vi "Set Controls.vi"(8 "error in (no error)":errorcluster, 9 "data values":variant[](array[variant]), 10 "control indexes":i32[](array[numeric]), 11 "VI Refnum in":refnum<vi>) -> (0 "error out":errorcluster)   [LabVIEW 2020, in "Msg.lvlib" / "Flex Msg.lvclass"]
doc: "Set control values using the 'Set Control Values by Index' method."
uses:
  Flex Msg.lvclass
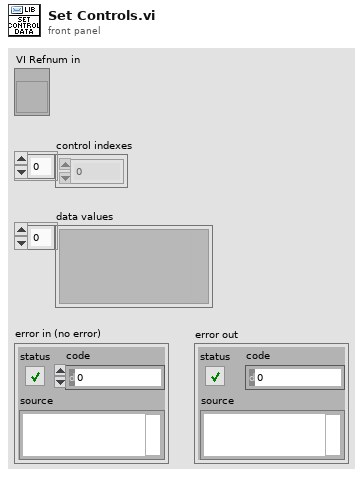
[diagram p1: front panel]
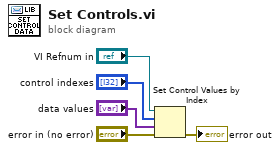
[diagram p0: block diagram]
diagram:
  n1 = Set Control Values by Index(0:"VI Refnum in", 1:"control indexes", 2:"data values", 3:"error in (no error)") -> (11:→"error out":errorcluster)
